vi "ReleaseDevice_8532.vi"(8 "Error In":errorcluster, 11 "task IN":T1={"Task Info"={"Accele Task"=[], "Simulate"=FALSE, "采样率"={"AISampleRate"=10123, "CouplingType"=10000, "Butter"=1000}, "Trig"={"PreTrigCNT"=0, "TriggerMode"=enum."中间触发", "TriggerSource"=enum."软件触发", "ATRTriggerChannel"=enum."通道0", "TriggerDir"=enum."下降沿触发", "TrigLevelVolt"=0.0, "bAvailableTrig"=FALSE}, "clock"={"EN"=FALSE, "clocksource"=enum."内部时钟", "outclocksource"=enum."Trig0"}, "delay(S)"=0.0}, "datain"={"nSegmentCount"=0, "chaneldataSize"=8192, "t0 in"=timestamp(0 s since 1904-01-01), "nsegmentsize"=0, "chanelcouter"=0}, "times"=0.0, "timer"=[], "\nen"=FALSE} {"Task Info"."采样率"."CouplingType" items=["直流耦合", "交流耦合"]}) -> (0 "Error Out":errorcluster, 3 "task OUT":T1={"Task Info"={"Accele Task"=[], "Simulate"=FALSE, "采样率"={"AISampleRate"=10123, "CouplingType"=10000, "Butter"=1000}, "Trig"={"PreTrigCNT"=0, "TriggerMode"=enum."中间触发", "TriggerSource"=enum."软件触发", "ATRTriggerChannel"=enum."通道0", "TriggerDir"=enum."下降沿触发", "TrigLevelVolt"=0.0, "bAvailableTrig"=FALSE}, "clock"={"EN"=FALSE, "clocksource"=enum."内部时钟", "outclocksource"=enum."Trig0"}, "delay(S)"=0.0}, "datain"={"nSegmentCount"=0, "chaneldataSize"=8192, "t0 in"=timestamp(0 s since 1904-01-01), "nsegmentsize"=0, "chanelcouter"=0}, "times"=0.0, "timer"=[], "\nen"=FALSE} {"Task Info"."采样率"."CouplingType" items=["直流耦合", "交流耦合"]})   [LabVIEW 2009]
uses:
  PCI8532_32.dll
  Ctrls/Acceleration Channel Config_Ctrls-某型振动实验台测试系统.ctl
  Ctrls/Sample Information.ctl
  Ctrls/Trig.ctl
  Ctrls/clock.ctl
  Ctrls/Task Info.ctl
  Ctrls/DATA info.ctl
  Ctrls/task.ctl
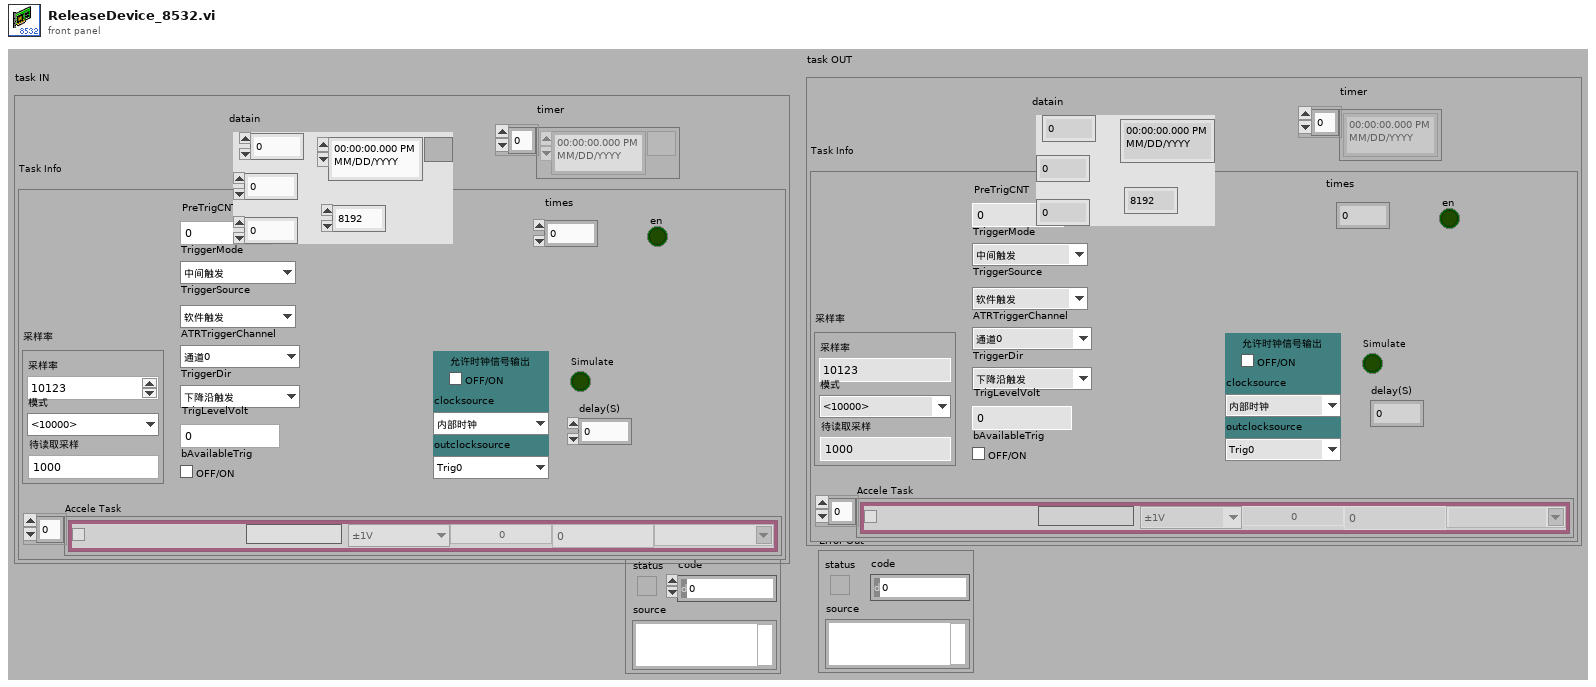
[diagram p1: front panel]
types:
  T1 = typedef "task.ctl" = cluster{"Task Info":T2, "datain":T7, "times":dbl, "timer":timestamp[], "\nen":bool}
  T2 = typedef "Task Info.ctl" = cluster{"Accele Task":T3[], "Simulate":bool, "采样率":T4, "Trig":T5, "clock":T6, "delay(S)":dbl}
  T3 = typedef "Acceleration Channel Config_Ctrls-某型振动实验台测试系统.ctl" = cluster{"Enable":bool, "Name":string, "range":enum16{"±1V", "±5V"}, "SensValue":dbl, "PhysicalName":string, "off":dbl, "Sensunits":string}
  T4 = typedef "Sample Information.ctl" = cluster{"AISampleRate":i32, "CouplingType":i32, "Butter":i32}
  T5 = typedef "Trig.ctl" = cluster{"PreTrigCNT":i32, "TriggerMode":enum16{"中间触发", "后触发", "预触发", "硬件延时触发"}, "TriggerSource":enum16{"软件触发", "DTR信号源", "ATR信号源", "Triger信号触发"}, "ATRTriggerChannel":enum16{"通道0", "通道1", "通道2", "通道3"}, "TriggerDir":enum16{"下降沿触发", "上升沿触发", "上下边没均触发"}, "TrigLevelVolt":sgl, "bAvailableTrig":bool}
  T6 = typedef "clock.ctl" = cluster{"EN":bool, "clocksource":enum16{"内部时钟", "外部时钟"}, "outclocksource":enum16{"Trig0", "Trig1", "Trig2", "Trig3", "Trig4", "Trig5", "Trig6", "Trig7", "PXI_STAR"}}
  T7 = typedef "DATA info.ctl" = cluster{"nSegmentCount":i32, "chaneldataSize":i32, "t0 in":timestamp, "nsegmentsize":i32, "chanelcouter":i32}
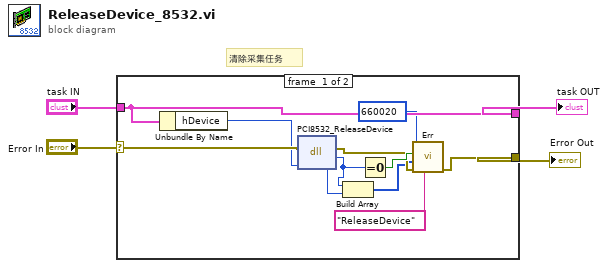
[diagram p0: block diagram]
diagram:
  # "清除采集任务"
  n1 = case shown="无错误" "Error In" {
    selector: "Error In" -> [w10 w17]
    tunnel: "task IN" -> [w15 w16]
    tunnel: [w14 w17] -> w2
    tunnel: [w15 w16] -> w1
    frame #0 {
      n2 = Unbundle By Name(w15) -> ("hDevice"=w9:i32)
      n3 = dll-call lib="PCI8532_32.dll" fn="PCI8532_ReleaseDevice" label="ReleaseDevice"(error in=w10, "hDevice"=w9) -> (error out=w8:errorcluster, "返回类型"=w7:i32, "hDevice"=w6:i32)  [unwired: 2 in, 1 out]
      n4 = Build Array(w7, w6) -> (w5:i32[])
      n5 = Equal To 0?(x=w7) -> (x = 0?=w12:bool)
      n6 = call "Err.vi"("source"="ReleaseDevice", "error in (no error)"=w8, "Par"=w5, "error?"=w12, "code"=660020) -> ("error out"=w14:errorcluster)  [unwired: 6 out]
    }
    frame #1 {
    }
  }
  "Error Out" <- w2
  "task OUT" <- w1
